vi "rad_UpdateAppVersionInInfoFile.vi"(8 "error in":errorcluster, 11 "Path to lvappimage.info":path) -> (0 "error out":errorcluster)   [LabVIEW 2016]
uses:
  rad_Globals.vi
  <vilib>/Utility/config.llb/Write Key (String).vi
  <vilib>/Utility/config.llb/NI_LVConfig.lvlib
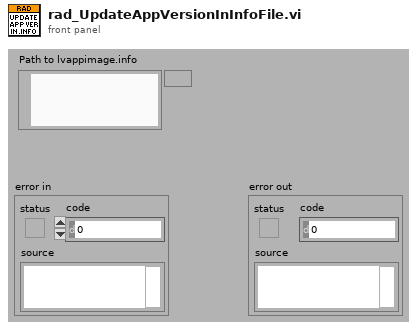
[diagram p1: front panel]
types:
  T1 = typedef "NI_LVConfig.lvlib/Config Data RefNum.ctl" = refnum<k1>
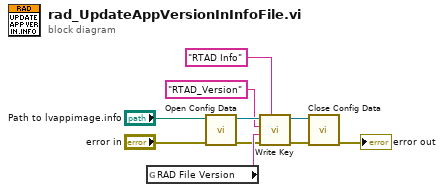
[diagram p0: block diagram]
diagram:
  n1 = global read "rad_Globals.vi" "RAD File Version"() -> (w10:string)
  n2 = call <vilib>:"Open Config Data.vi"("error in (no error)"="error in", "configuration file path"="Path to lvappimage.info") -> ("error out"=w6:errorcluster, "refnum"=w4:T1)  [unwired: 7 in, 1 out]
  n3 = call-poly <vilib>:"Write Key.vi"("section"="RTAD Info", "error in (no error)"=w6, "value"=w10, "key"="RTAD_Version", "refnum"=w4) -> ("error out"=w7:errorcluster, "refnum out"=w2:T1)  [unwired: 4 in, 1 out]
  n4 = call <vilib>:"Close Config Data.vi"("error in (no error)"=w7, "refnum"=w2) -> ("error out"=→"error out":errorcluster)  [unwired: 8 in, 1 out]
